vi "GPIO Read.vi"(8 "error in (no error)":errorcluster, 11 "Rpi.GPIO":T1=7 items=["GPIO2 (P1_3-SDA)"=2, "GPIO3 (P1_5-SCL)"=3, "GPIO4 (P1_7)"=4, "GPIO17 (P1_11)"=17, "GPIO27 (P1_13)"=27, "GPIO22 (P1_15)"=22, "GPIO10 (P1_19-MOSI)"=10, "GPIO9 (P1_21-MISO)"=9, "GPIO11 (P1_23SCLK)"=11, "GPIO5 (P1_29)"=5, "GPIO6 (P1_31)"=6, "GPIO13 (P1_33-PWM1)"=13, "GPIO19 (P1_35)"=19, "GPIO26 (P1_37)"=26, "GPIO14 (P1_8-UART-Tx)"=14, "GPIO15 (P1_10-UART-Rx)"=15, "GPIO18 (P1_12)"=18, "GPIO23 (P1_16)"=23, "GPIO24 (P1_18)"=24, "GPIO25 (P1_22)"=25, "GPIO8 (P1_24-CE0)"=8, "GPIO7 (P1_26-CE1)"=7, "GPIO12 (P1_32-PWM0)"=12, "GPIO16 (P1_36)"=16, "GPIO20 (P1_38)"=20, "GPIO21 (P1_40)"=21]) -> (0 "error out":errorcluster, 3 "status":i32)   [LabVIEW 2014, in "QwaveSys Raspberry Pi Library.lvlib"]
uses:
  QwaveSys Raspberry Pi Library.lvlib
  RPi GPIO.ctl
panel:
  out "standard output":string
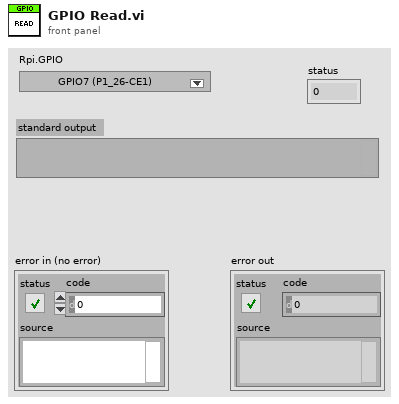
[diagram p1: front panel]
types:
  T1 = typedef "QwaveSys Raspberry Pi Library.lvlib/RPi GPIO.ctl" = u8
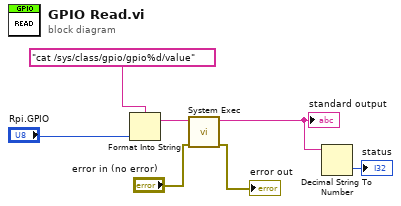
[diagram p0: block diagram]
diagram:
  n1 = Format Into String(format string="cat /sys/class/gpio/gpio%d/value" ("command line"), "Rpi.GPIO") -> (resulting string=w7:string)  [unwired: 2 in, 1 out]
  n2 = call <vilib>:"System Exec.vi"("error in (no error)"="error in (no error)", "command line"=w7) -> ("error out"=→"error out":errorcluster, "standard output"=w5:string)  [unwired: 6 in, 2 out]
  "standard output" <- w5
  n3 = Decimal String To Number(string=w5) -> (number=→"status":i32)  [unwired: 2 in, 1 out]
